vi "QX_StopDaq.vi"(8 "Error in":errorcluster, 11 "DaqMeasurement":refnum<k24>) -> (0 "Error out":errorcluster)   [LabVIEW 2016]
doc: "Stops data acquisition of all devices that take part in the measurement"
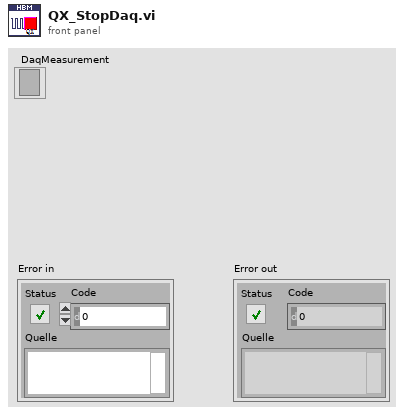
[diagram p1: front panel]
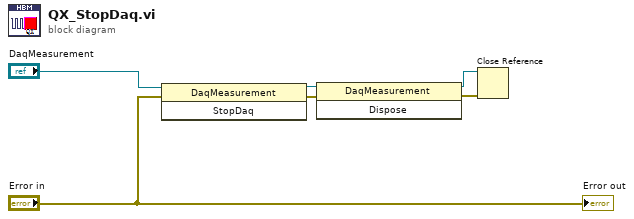
[diagram p0: block diagram]
diagram:
  n1 = invoke on="Methodenknoten" class="DaqMeasurement" method="StopDaq"(reference="DaqMeasurement", error in="Error in") -> (reference out=w4:refnum<k24>, error out=w5:errorcluster)  [unwired: 1 in, 1 out]
  n2 = invoke on="Methodenknoten" class="DaqMeasurement" method="Dispose"(reference=w4, error in=w5) -> (reference out=w2:refnum<k24>, error out=w3:errorcluster)  [unwired: 1 in, 1 out]
  n3 = Close Reference(reference=w2, error in (no error)=w3) -> ()  [unwired: 1 out]
  "Error out" <- "Error in"
